vi "Server Single Connection.vi"() -> ()   [LabVIEW 2021]
doc: "This WebSockets API example VI acts as a server for an incoming websockets connection. Receives/sends string data to the connected client."
uses:
  WebSockets/WebSocket/WebSocket.lvclass/WebSocket.ctl
  WebSockets/WebSocket Server/WebSocket Server.lvclass/WebSocket Server.ctl
  WebSockets/WebSocket/Read Return Headers.vi
  WebSockets/WebSocket Server/Read Request URI.vi
  WebSockets/WebSocket Server/WebSocket Server.lvclass
  D:/my_projects/projects/Algorithms/Labview/21/WebSockets/Source/WebSockets/WebSocket/WebSocket.lvclass
  Sockets/VISA TCP Listener/VISA TCP Listener.lvclass
panel:
  out "Request URI":string
  out "HTTP Headers":variant
  in  "Stop":bool
  out "Received Data":string
  in  "Send":bool
  in  "Data":string
  # "WebSockets Server Example"
  # "This VI is a simple example of sending/receiving data using WebSockets.\nIt waits for a single incoming WebSockets connection on Port 6123 and\nthen displays incoming string data. Strings can also be sent back to the client.\n\nInstructions for use:\n1) Run this VI\n2) Open the index.html file located in the examples folder or the 'Client Single Connection' example or deploy the 'Test Client' web service and visiting the web service URL\n3) The index.html will display the status of the connection and once established, data can be sent/received from either this VI or the index.html file.\n\nNote: For Microsoft Edge, you may need to access the index.html file by first deploying the 'Test Client' Web Service, executing \"CheckNetIsolation LoopbackExempt -a -n=Microsoft.MicrosoftEdge_8wekyb3d8bbwe\" to enable WebSockets on a loopback and then visiting http://localhost:<web service port>/index.html"
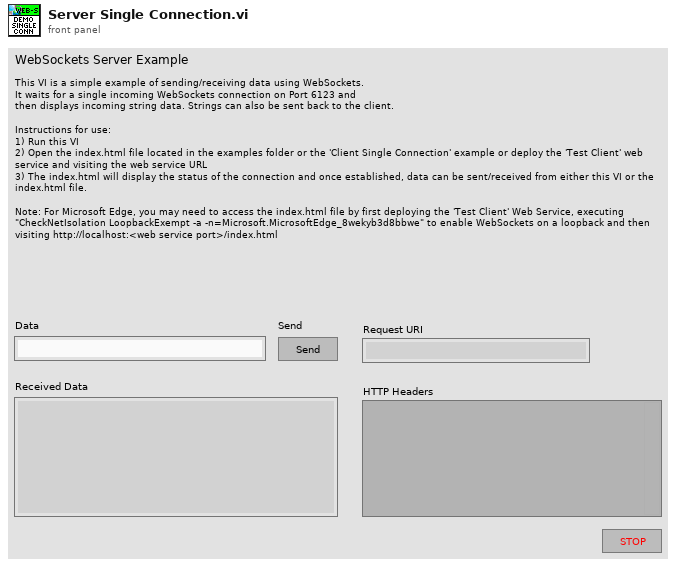
[diagram p1: front panel]
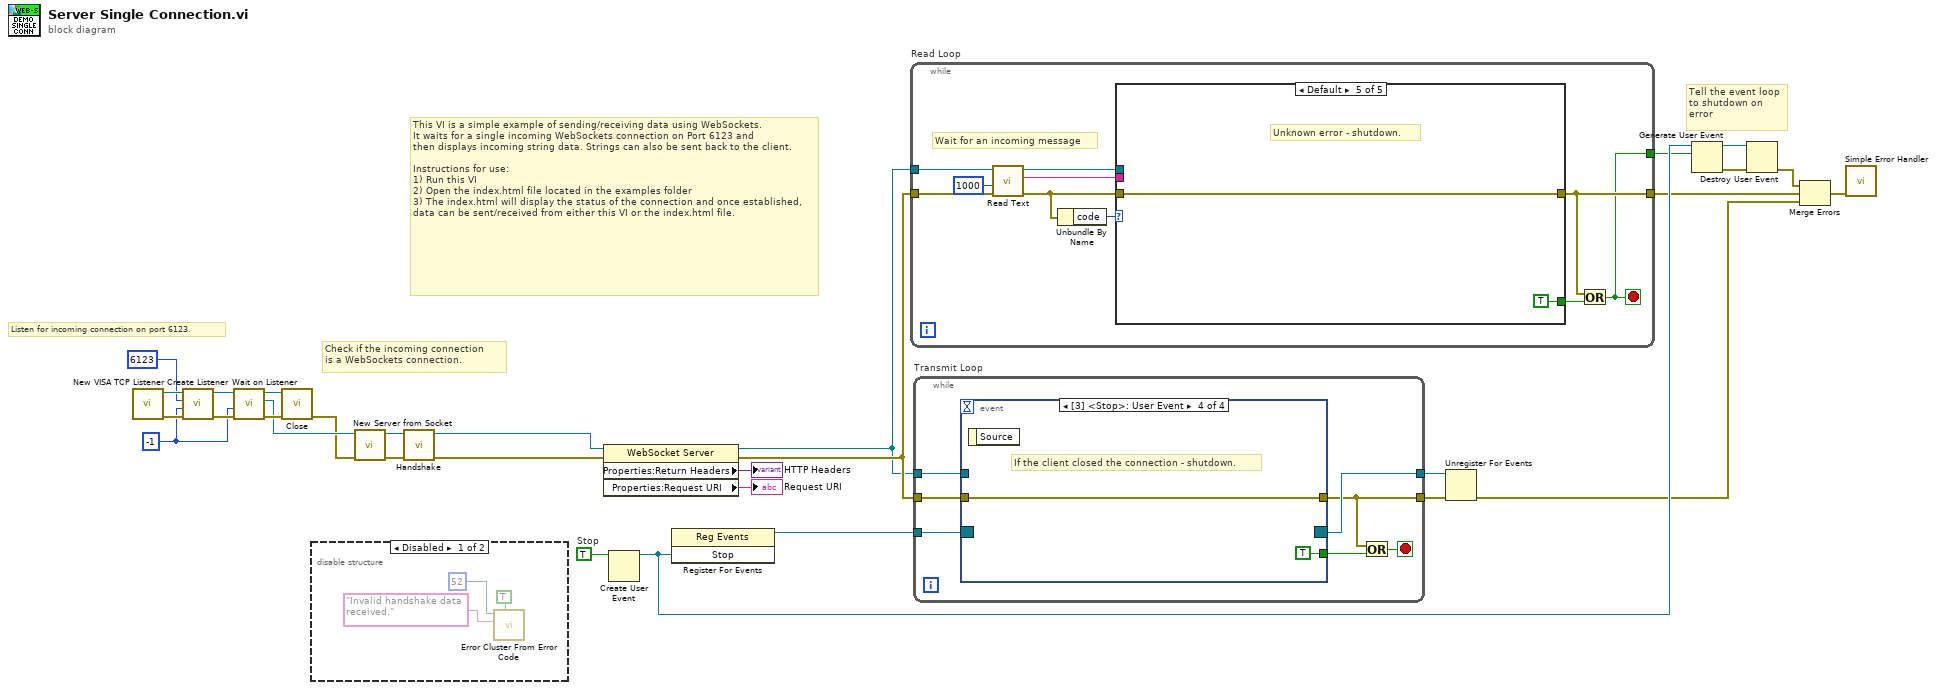
[diagram p0: block diagram]
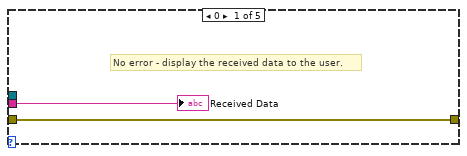
[diagram p3: hidden frame]
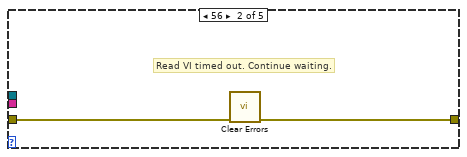
[diagram p4: hidden frame]
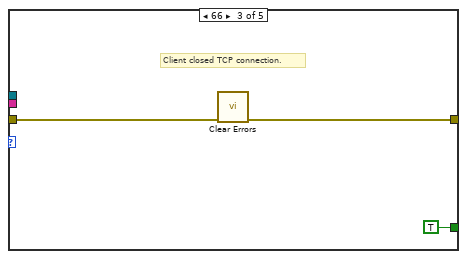
[diagram p5: hidden frame]
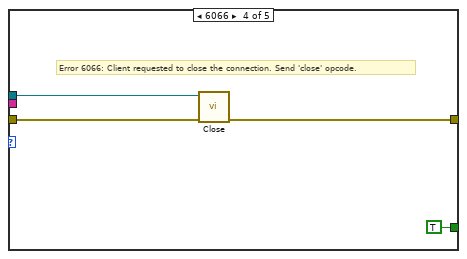
[diagram p6: hidden frame]
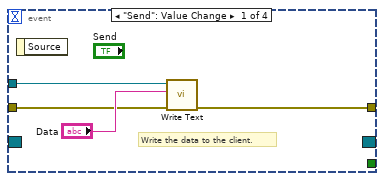
[diagram p7: hidden frame]
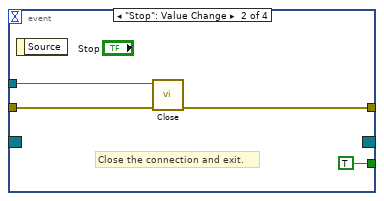
[diagram p8: hidden frame]
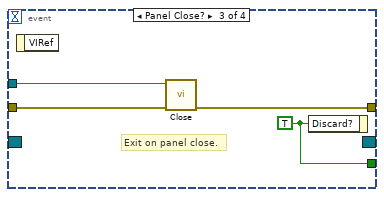
[diagram p9: hidden frame]
diagram:
  w29 = TRUE  # Stop
  w5 = -1 ("timeout ms (25000)")
  # "Tell the event loop to shutdown on error"
  # "This VI is a simple example of sending/receiving data using WebSockets.\nIt waits for a single incoming WebSockets connection on Port 6123 and\nthen displays incoming string data. Strings can also be sent back to the client.\n\nInstructions for use:\n1) Run this VI\n2) Open the index.html file located in the examples folder\n3) The index.html will display the status of the connection and once established, data can be sent/received from either this VI or the index.html file."
  # "Check if the incoming connection\nis a WebSockets connection."
  # "Listen for incoming connection on port 6123."
  n1 = call "New VISA TCP Listener.vi"() -> ("error out"=w11:errorcluster, "VISA TCP Listener out"=w12:refnum<class "VISA TCP Listener.lvclass">)  [unwired: 10 in]
  n2 = call-dynamic "Create Listener.vi"("error in (no error)"=w11, "timeout ms (5000)"=w5, "Port"=u16 6123 ("port"), "VISA TCP Listener in"=w12) -> ("error out"=w9:errorcluster, "VISA TCP Listener out"=w7:refnum<class "VISA TCP Listener.lvclass">)  [unwired: 6 in]
  n3 = call-dynamic "Wait on Listener.vi"("error in (no error)"=w9, "timeout ms (5000)"=w5, "VISA TCP Listener in"=w7) -> ("error out"=w10:errorcluster, "Socket out"=w4:refnum<class "Socket.lvclass">, "VISA TCP Listener out"=w8:refnum<class "VISA TCP Listener.lvclass">)  [unwired: 6 in]
  n4 = call-dynamic "Close.vi"("error in (no error)"=w10, "VISA TCP Listener in"=w8) -> ("error out"=w3:errorcluster)  [unwired: 9 in]
  n5 = disable-structure shown="Disabled" {
    frame Disabled {
      n6 = call <vilib>:"Error Cluster From Error Code.vi"("show call chain? (False)"=TRUE, "error message (\"\")"="Invalid handshake data received." ("error message (\"\")"), "error code (0)"=52) -> ()  [unwired: 6 in, 1 out]
    }
    frame Enabled {
    }
  }
  n7 = call "New Server from Socket.vi"("error in (no error)"=w3, "Socket"=w4) -> ("error out"=w17:errorcluster, "WebSocket Server out"=w18:refnum<class "WebSocket Server.lvclass">)  [unwired: 8 in]
  n8 = call-dynamic "Handshake.vi"("error in (no error)"=w17, "WebSocket Connection in"=w18) -> ("error out"=w1:errorcluster, "WebSocket Connection out"=w2:refnum<class "WebSocket Server.lvclass">)  [unwired: 8 in]
  n9 = property class="WebSocket Server"(reference=w2, error in=w1) -> (reference out=w15:refnum<class "WebSocket Server.lvclass">, error out=w16:errorcluster, "Properties:Return Headers"=→"HTTP Headers":variant, "Properties:Request URI"=→"Request URI":string)
  n10 = Create User Event(user event datatype=w29) -> (user event=w27:refnum<user-event>)  [unwired: 1 in, 1 out]
  n11 = register-events(w27) -> (reference out=w30:refnum<event-registration>)  [unwired: 2 in, 1 out]
  n12 = while "Read Loop" {
    tunnel: w15 -> [w43]
    tunnel: [w34] -> w26
    tunnel: [w36] -> w20
    tunnel: w16 -> [w37]
    stop <- w34 stop-if-true
    # "Wait for an incoming message"
    n13 = call-dynamic "Read Text.vi"("error in (no error)"=w37, "timeout ms (5000)"=1000 ("timeout ms (25000)"), "WebSocket in"=w43) -> ("error out"=w38:errorcluster, "Data"=w40:string, "WebSocket out"=w39:refnum<class "WebSocket Server.lvclass">)  [unwired: 6 in]
    n14 = Unbundle By Name(w38) -> ("code"=w41:i32)
    n15 = case shown="Default" w41 {
      tunnel: w40 -> [w45 _ _ _ _]
      tunnel: [_ _ TRUE TRUE TRUE] -> w35
      tunnel: w39 -> [_ _ _ w54 _]
      tunnel: w38 -> [w44 w47 w49 w52 w55]
      tunnel: [w44 w46 w48 w51 w55] -> w36
      frame 0 {
        # "No error - display the received data to the user."
        "Received Data" <- w45
      }
      frame 56 {
        # "Read VI timed out. Continue waiting."
        n16 = call <vilib>:"Clear Errors.vi"("error in (no error)"=w47) -> ("error out"=w46:errorcluster)  [unwired: 5 in, 1 out]
      }
      frame 66 {
        # "Client closed TCP connection."
        n17 = call <vilib>:"Clear Errors.vi"("error in (no error)"=w49) -> ("error out"=w48:errorcluster)  [unwired: 5 in, 1 out]
      }
      frame 6066 {
        # "Error 6066: Client requested to close the connection. Send 'close' opcode."
        n18 = call-dynamic "Close.vi"("error in (no error)"=w52, "WebSocket in"=w54) -> ("error out"=w51:errorcluster)  [unwired: 8 in, 1 out]
      }
      frame Default {
        # "Unknown error - shutdown."
      }
    }
    n19 = Or(x=w36, y=w35) -> (x .or. y?=w34:bool)
  }
  n20 = while "Transmit Loop" {
    tunnel: w15 -> [w63]
    tunnel: w30 -> [w62]
    tunnel: [w61] -> w28
    tunnel: [w57] -> w21
    tunnel: w16 -> [w60]
    stop <- w58 stop-if-true
    n21 = event shown="[3] <Stop>: User Event" {
      selector: w62 -> [_ _ _ _]
      dyn-events: [_ _ _ _] -> w61
      timeout: _ -> [_ _ _ _]
      tunnel: w63 -> [w67 w70 w75 _]
      tunnel: [_ TRUE w74 TRUE] -> w59
      tunnel: [w64 w69 w73 w76] -> w57
      tunnel: w60 -> [w65 w68 w72 w76]
      event "Send": Value Change {
        # "Write the data to the client."
        n22 = event-data() -> ()  [unwired: 1 in, 1 out]
        n23 = call-dynamic "Write Text.vi"("error in (no error)"=w65, "String Data"="Data", "WebSocket in"=w67) -> ("error out"=w64:errorcluster)  [unwired: 7 in, 1 out]
      }
      event "Stop": Value Change {
        # "Close the connection and exit."
        n24 = event-data() -> ()  [unwired: 1 in, 1 out]
        n25 = call-dynamic "Close.vi"("error in (no error)"=w68, "WebSocket in"=w70) -> ("error out"=w69:errorcluster)  [unwired: 8 in, 1 out]
      }
      event Panel Close? {
        w74 = TRUE ("Discard?")
        # "Exit on panel close."
        n26 = event-data() -> ()  [unwired: 1 in, 1 out]
        n27 = call-dynamic "Close.vi"("error in (no error)"=w72, "WebSocket in"=w75) -> ("error out"=w73:errorcluster)  [unwired: 8 in, 1 out]
        n28 = event-data("Discard?"=w74) -> ()  [unwired: 1 in, 1 out]
      }
      event User Event {
        # "If the client closed the connection - shutdown."
        n29 = event-data() -> ()  [unwired: 1 in, 1 out]
      }
    }
    n30 = Or(x=w57, y=w59) -> (x .or. y?=w58:bool)
  }
  n31 = Unregister For Events(event registration refnum=w28, error in=w21) -> (error out=w19:errorcluster)
  n32 = Generate User Event(user event=w27, event data cluster=w26) -> (user event out=w25:refnum<user-event>, error out=w24:errorcluster)  [unwired: 2 in]
  n33 = Destroy User Event(user event=w25, error in=w24) -> (error out=w23:errorcluster)
  n34 = Merge Errors(w23, w20, w19) -> (w22:errorcluster)
  n35 = call <vilib>:"Simple Error Handler.vi"("error in (no error)"=w22) -> ()  [unwired: 4 in, 5 out]
